vi "Parse Header.vi"(0 "header in":u8 format="%.0x") -> (4 "write":bool, 6 "address":u8 format="%.0x")   [LabVIEW 2013, in "DIO SPI User Library.lvlib"]
doc: "Converts byte into read/write command and address. This VI could be updated to support any header format."
uses:
  DIO SPI User Library.lvlib
panel:
  # "Converts byte into read/write command and address. This VI could be updated to support any header format."
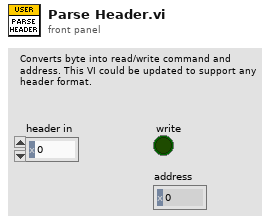
[diagram p1: front panel]
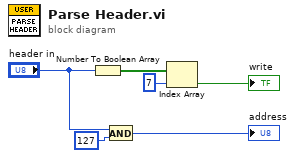
[diagram p0: block diagram]
diagram:
  n1 = Number To Boolean Array(number="header in") -> (Boolean array=w3:bool[])
  n2 = And(x="header in", y=u8 127 ("Header")) -> (x .and. y?=→"address":u8)
  n3 = Index Array(array=w3, index=7) -> (element=→"write":bool)
